vi "Status Update Impl.vi"(8 "error in (no error)":errorcluster, 11 "Alltesta Autosampler in":refnum<class "Alltesta Autosampler.lvclass">) -> (0 "error out":errorcluster, 2 "Autosampler Status":T1, 3 "Alltesta Autosampler out":refnum<class "Alltesta Autosampler.lvclass">)   [LabVIEW 2023, in "Alltesta Autosampler.lvlib" / "Alltesta Autosampler.lvclass"]
uses:
  Alltesta Autosampler.lvclass
  Autosampler/Autosampler Status.ctl
  Autosampler/Autosampler State.ctl
  Alltesta Autosampler.lvclass/Alltesta Autosampler.ctl
  Alltesta Autosampler.lvlib
  Autosampler/Autosampler.lvlib
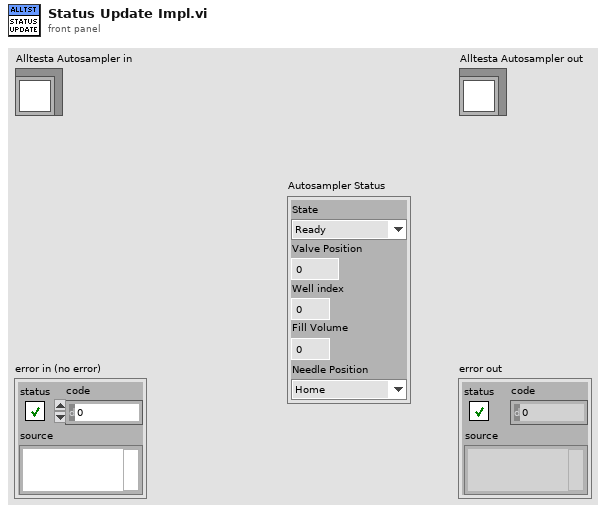
[diagram p1: front panel]
types:
  T1 = typedef "Autosampler.lvlib/Autosampler Status.ctl" = cluster{"State":T2, "Valve Position":u16, "Well index":u16, "Fill Volume":u16, "Needle Position":enum16{"Home", "Well", "Wash Port"}}
  T2 = typedef "Autosampler.lvlib/Autosampler State.ctl" = enum16{"Ready", "Injection", "Washing", "Shaking", "Getting Ready", "Error"}
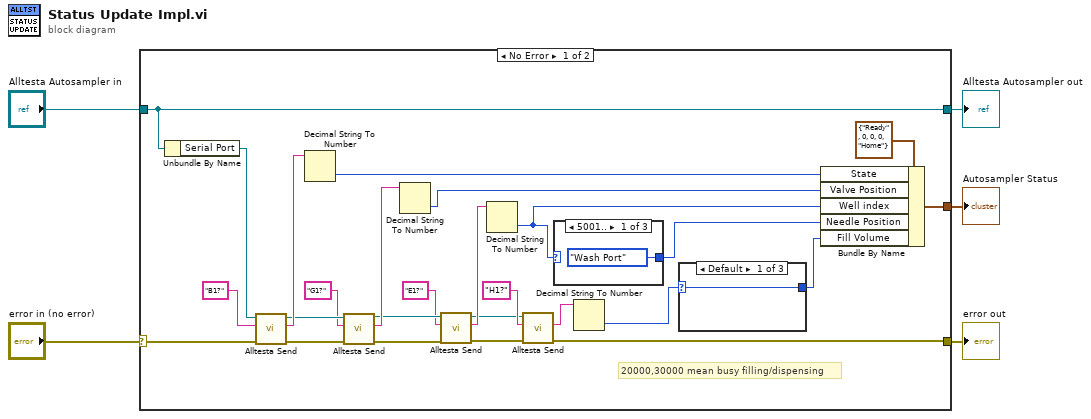
[diagram p0: block diagram]
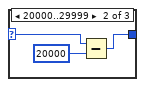
[diagram p2: hidden frame]
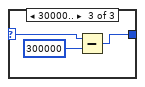
[diagram p3: hidden frame]
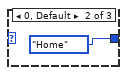
[diagram p4: hidden frame]
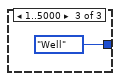
[diagram p5: hidden frame]
diagram:
  n1 = case shown="No Error" "error in (no error)" {
    selector: "error in (no error)" -> [w31 w43]
    tunnel: [w10 w43] -> w4
    tunnel: "Alltesta Autosampler in" -> [w30 w42]
    tunnel: [w30 w42] -> w2
    tunnel: [w26 _] -> w1
    frame No Error {
      # "20000,30000 mean busy filling/dispensing"
      n2 = Unbundle By Name(w30) -> ("Serial Port"=w29:refnum<visa-resource-name>)
      n3 = call "Alltesta Send.vi"("error in (no error)"=w31, "Command"="B1?", "Serial Port in"=w29) -> ("error out"=w23:errorcluster, "Response"=w25:string, "Serial Port out"=w22:refnum<visa-resource-name>)  [unwired: 6 in]
      n4 = Decimal String To Number(string=w25) -> (number=w24:i32)  [unwired: 2 in, 1 out]
      n5 = call "Alltesta Send.vi"("error in (no error)"=w23, "Command"="G1?", "Serial Port in"=w22) -> ("error out"=w19:errorcluster, "Response"=w20:string, "Serial Port out"=w18:refnum<visa-resource-name>)  [unwired: 6 in]
      n6 = Decimal String To Number(string=w20) -> (number=w15:i32)  [unwired: 2 in, 1 out]
      n7 = call "Alltesta Send.vi"("error in (no error)"=w19, "Command"="E1?", "Serial Port in"=w18) -> ("error out"=w13:errorcluster, "Response"=w16:string, "Serial Port out"=w12:refnum<visa-resource-name>)  [unwired: 6 in]
      n8 = Decimal String To Number(string=w16) -> (number=w9:i32)  [unwired: 2 in, 1 out]
      n9 = call "Alltesta Send.vi"("error in (no error)"=w13, "Command"="H1?", "Serial Port in"=w12) -> ("error out"=w10:errorcluster, "Response"=w11:string)  [unwired: 6 in, 1 out]
      n10 = case shown="5001.." w9 {
        tunnel: [enum16{"Home", "Well", "Wash Port"}."Wash Port" ("Needle Position") enum16{"Home", "Well", "Wash Port"}."Home" ("Needle Position") enum16{"Home", "Well", "Wash Port"}."Well" ("Needle Position")] -> w8
        frame 5001.. {
        }
        frame 0, Default {
        }
        frame 1..5000 {
        }
      }
      n11 = Decimal String To Number(string=w11) -> (number=w7:i32)  [unwired: 2 in, 1 out]
      n12 = case shown="Default" w7 {
        selector: w7 -> [w32 w34 w37]
        tunnel: [w32 w33 w38] -> w6
        frame Default {
        }
        frame 20000..29999 {
          n13 = Subtract(x=w34, y=20000) -> (x-y=w33:i32)
        }
        frame 30000.. {
          n14 = Subtract(x=w37, y=300000) -> (x-y=w38:i32)
        }
      }
      n15 = Bundle By Name(cluster=T1 {"State"=enum."Ready", "Valve Position"=0, "Well index"=0, "Fill Volume"=0, "Needle Position"=enum."Home"} ("Autosampler Status"), "State"=w24, "Valve Position"=w15, "Well index"=w9, "Needle Position"=w8, "Fill Volume"=w6) -> (w26:T1)
    }
    frame Error {
    }
  }
  "error out" <- w4
  "Alltesta Autosampler out" <- w2
  "Autosampler Status" <- w1
